vi "Get Strings from Ref.vi"(8 "error in (no error)":errorcluster, 9 "Label Prefix":string, 10 "GObj Refnum in":refnum<vi>, 11 "ArrayConstant in":refnum<class "ArrayConstant.lvclass">) -> (0 "error out":errorcluster, 1 "Valid?":bool, 2 "GObj Refnum out":refnum<vi>, 3 "ArrayConstant out":refnum<class "ArrayConstant.lvclass">, 4 "GObj Name":string)   [LabVIEW 2013, in "SET Project Data.lvlib" / "ArrayConstant.lvclass"]
uses:
  ArrayConstant.lvclass
  GObject/GObject.lvclass/GObject.ctl
  GObject/Write Label.vi
  GObject/Write UID.vi
  GObject/Write ClassName.vi
  GObject/GObject.lvclass
  SET Project Data.lvlib
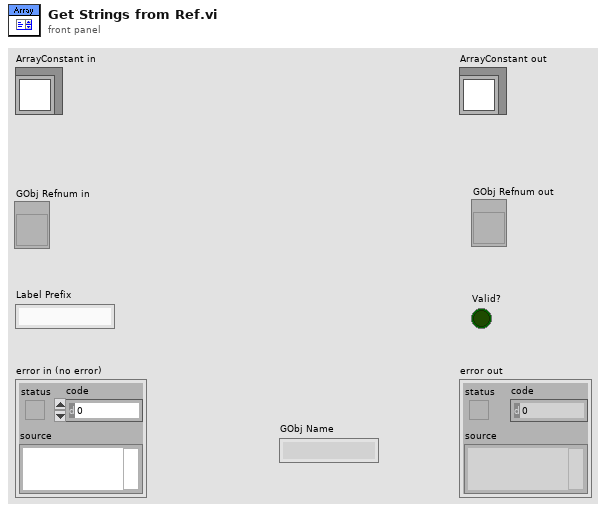
[diagram p1: front panel]
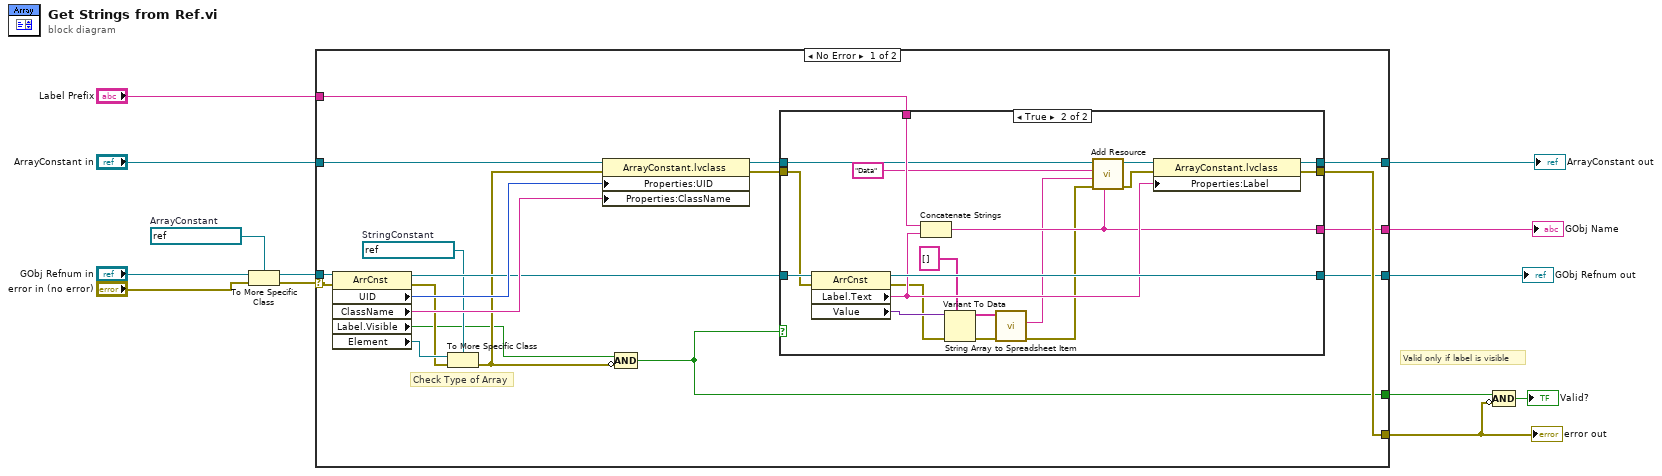
[diagram p0: block diagram]
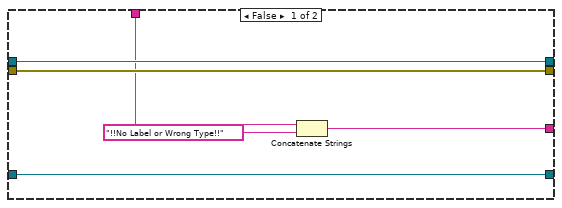
[diagram p2: hidden frame]
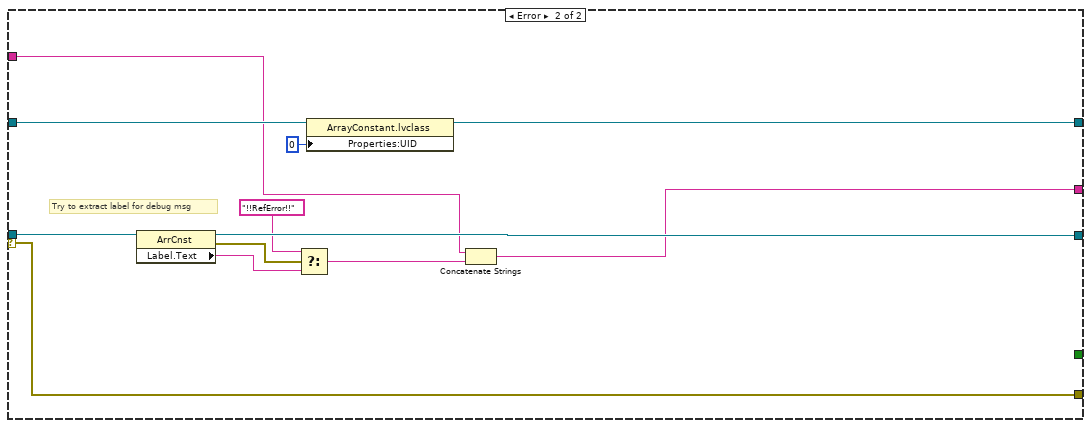
[diagram p3: hidden frame]
diagram:
  w4 = refnum<vi> refnum  # ArrayConstant
  # "Valid only if label is visible"
  n1 = To More Specific Class(target class=w4, reference="GObj Refnum in", error in="error in (no error)") -> (specific class reference=w12:refnum<vi>, error out=w11:errorcluster)
  n2 = case shown="No Error" w11 {
    selector: w11 -> [w25 w68]
    tunnel: w12 -> [w31 w64]
    tunnel: [w22 w63] -> w7
    tunnel: [w23 w68] -> w5
    tunnel: "ArrayConstant in" -> [w32 w67]
    tunnel: [w27 w65] -> w9
    tunnel: "Label Prefix" -> [w21 w58]
    tunnel: [w14 _] -> w13
    tunnel: [w20 w62] -> w8
    frame No Error {
      w17 = refnum<vi> refnum  # StringConstant
      # "Check Type of Array"
      n3 = property class="ArrCnst"(reference=w31, error in=w25) -> (reference out=w26:refnum<vi>, error out=w18:errorcluster, "UID"=w30:i32, "ClassName"=w29:string, "Label.Visible"=w15:bool, "Element"=w19:refnum<vi>)
      n4 = To More Specific Class(target class=w17, reference=w19, error in=w18) -> (error out=w16:errorcluster)  [unwired: 1 out]
      n5 = property class="ArrayConstant.lvclass"(reference=w32, error in=w16, "Properties:UID"=w30, "Properties:ClassName"=w29) -> (reference out=w28:refnum<class "ArrayConstant.lvclass">, error out=w24:errorcluster)
      n6 = Compound Arithmetic op=AND(w15, invert w16) -> (w14:bool)
      n7 = case shown="True" w14 {
        tunnel: w28 -> [w38 w50]
        tunnel: [w38 w56] -> w27
        tunnel: w26 -> [w36 w55]
        tunnel: w24 -> [w37 w54]
        tunnel: [w37 w53] -> w23
        tunnel: [w36 w52] -> w22
        tunnel: w21 -> [w35 w51]
        tunnel: [w33 w45] -> w20
        frame False {
          n8 = Concatenate Strings(w35, "!!No Label or Wrong Type!!") -> (w33:string)
        }
        frame True {
          n9 = property class="ArrCnst"(reference=w55, error in=w54) -> (reference out=w52:refnum<vi>, error out=w40:errorcluster, "Label.Text"=w46:string, "Value"=w44:variant)
          n10 = Concatenate Strings(w51, w46) -> (w45:string)
          n11 = Variant To Data(error in=w40, type=string[] [], Variant=w44) -> (data=w42:string[], error out=w39:errorcluster)
          n12 = call "String Array to Spreadsheet Item.vi"("Strings [] (ASCII)"=w42) -> ("Spreadsheet Item (ASCII)"=w41:string)  [unwired: 10 in]
          n13 = call "Add Resource.vi"("TagPrefix"=w45, "error in (no error)"=w39, "ItemText"=w41, "ItemName"="Data" ("name"), "GObject in"=w50) -> ("error out"=w47:errorcluster, "GObject out"=w49:refnum<class "ArrayConstant.lvclass">)  [unwired: 5 in]
          n14 = property class="ArrayConstant.lvclass"(reference=w49, error in=w47, "Properties:Label"=w46) -> (reference out=w56:refnum<class "ArrayConstant.lvclass">, error out=w53:errorcluster)
        }
      }
    }
    frame Error {
      # "Try to extract label for debug msg"
      n15 = property class="ArrCnst"(reference=w64) -> (reference out=w63:refnum<vi>, error out=w61:errorcluster, "Label.Text"=w59:string)  [unwired: 1 in]
      n16 = Select(t="!!RefError!!" ("Label.Text"), s=w61, f=w59) -> (s? t:f=w57:string)
      n17 = property class="ArrayConstant.lvclass"(reference=w67, "Properties:UID"=0 ("UID")) -> (reference out=w65:refnum<class "ArrayConstant.lvclass">)  [unwired: 1 in, 1 out]
      n18 = Concatenate Strings(w58, w57) -> (w62:string)
    }
  }
  "error out" <- w5
  "ArrayConstant out" <- w9
  "GObj Refnum out" <- w7
  "GObj Name" <- w8
  n19 = Compound Arithmetic op=AND(w13, invert w5) -> (→"Valid?":bool)
